vi "Read Parameters.vi"(8 "error in (no error)":errorcluster, 11 "Build Job in":refnum<class "Build Job.lvclass">) -> (0 "error out":errorcluster, 2 "Parameters":variant, 3 "Build Job out":refnum<class "Build Job.lvclass">)   [LabVIEW 2014, in "Build Job.lvclass"]
uses:
  Build Job.lvclass
  Build Job.lvclass/Build Job.ctl
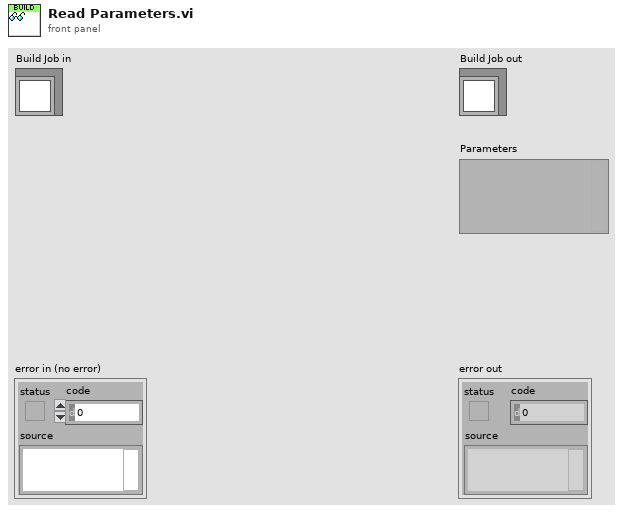
[diagram p1: front panel]
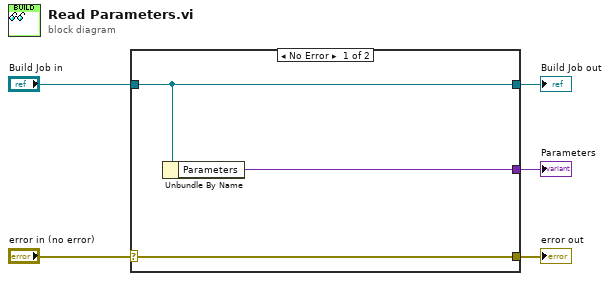
[diagram p0: block diagram]
diagram:
  n1 = case shown="No Error" "error in (no error)" {
    selector: "error in (no error)" -> [w8 w9]
    tunnel: [w8 w9] -> w4
    tunnel: [w7 w10] -> w2
    tunnel: "Build Job in" -> [w7 w10]
    tunnel: [w6 _] -> w1
    frame No Error {
      n2 = Unbundle By Name(w7) -> ("Parameters"=w6:variant)
    }
    frame Error {
    }
  }
  "error out" <- w4
  "Build Job out" <- w2
  "Parameters" <- w1
